vi "Read Data File.lvclass.vi"(8 "error in (no error)":errorcluster, 11 "Data Loader in":refnum<class "Data Loader.lvclass">) -> (0 "error out":errorcluster, 2 "Abstruct Data Type.lvclass":refnum<class "Abstruct Data Type.lvclass">, 3 "Data Loader out":refnum<class "Data Loader.lvclass">)   [LabVIEW 2020, in "Data Loader.lvlib" / "Data Loader.lvclass"]
uses:
  Data Loader.lvclass
  Data Types/Abstrut Data/Abstruct Data Type.lvclass
  Data Loader.lvclass/Data Loader.ctl
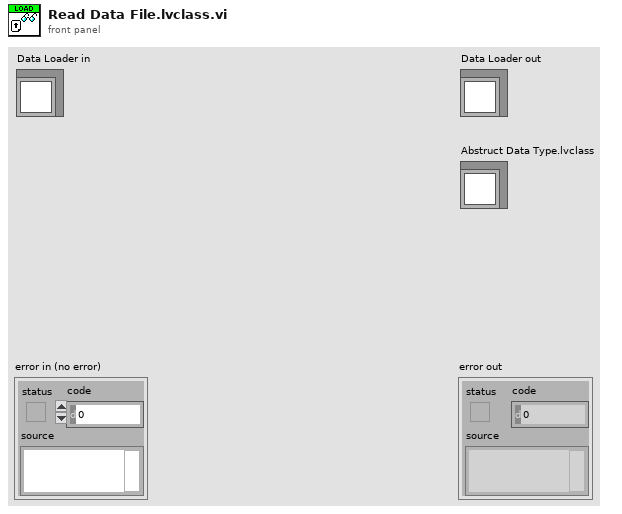
[diagram p1: front panel]
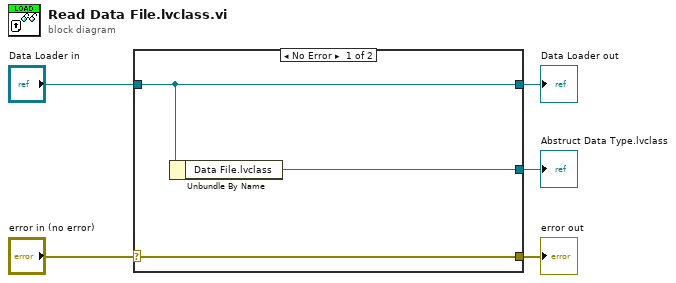
[diagram p0: block diagram]
diagram:
  n1 = case shown="No Error" "error in (no error)" {
    selector: "error in (no error)" -> [w8 w9]
    tunnel: [w8 w9] -> w4
    tunnel: [w7 w10] -> w2
    tunnel: "Data Loader in" -> [w7 w10]
    tunnel: [w6 _] -> w1
    frame No Error {
      n2 = Unbundle By Name(w7) -> ("Data File.lvclass"=w6:refnum<class "Abstruct Data Type.lvclass">)
    }
    frame Error {
    }
  }
  "error out" <- w4
  "Data Loader out" <- w2
  "Abstruct Data Type.lvclass" <- w1
